vi "WS1050 CAPDAC Setting Updated.vi"(6 "DUT Mask Mode (All)":T1=enum."All", 8 "error in":errorcluster, 9 "C3 Cap DAC":u8=128 caption="B Data In" format="0x%02x", 10 "C2 Cap DAC":u8=128 caption="B Data In" format="0x%02x", 11 "C1 Cap DAC":u8=128 caption="B Data In" format="0x%02x") -> (0 "error out":errorcluster)   [LabVIEW 2012]
uses:
  WS_VCAP Driver 029/Source/WSVCAP Shell/Type Defs/WSVCAP SHL I2C DUT Mask Mode Enum.ctl
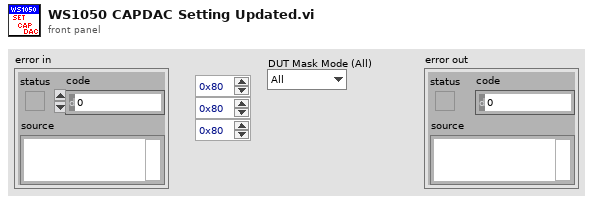
[diagram p1: front panel]
types:
  T1 = typedef "WSVCAP SHL I2C DUT Mask Mode Enum.ctl" = enum16{"Custom", "C1", "C2", "C3", "All"}
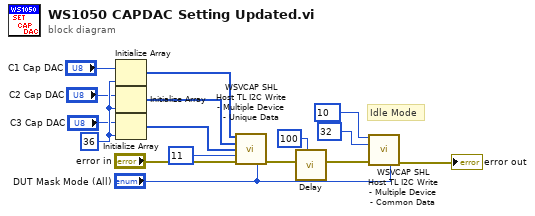
[diagram p0: block diagram]
diagram:
  w16 = 36 ("dimension size")
  # "Idle Mode"
  n1 = Initialize Array("C1 Cap DAC", w16) -> (w2:u8[])
  n2 = Initialize Array("C2 Cap DAC", w16) -> (w3:u8[])
  n3 = Initialize Array("C3 Cap DAC", w16) -> (w1:u8[])
  n4 = call "WSVCAP SHL Host TL I2C Write - Multiple Device - Unique Data.vi"("C1 Data"=w2, "C2 Data"=w3, "C3 Data"=w1, "Sub Address"=u8 11, "error in"="error in", "DUT Mask Mode (All)"="DUT Mask Mode (All)") -> ("error out"=w8:errorcluster)  [unwired: 9 in]
  n5 = call "Delay.vi"("milliseconds to wait"=u32 100, "error in (no error)"=w8) -> ("error out"=w4:errorcluster)  [unwired: 9 in]
  n6 = call "WSVCAP SHL Host TL I2C Write - Multiple Device - Common Data.vi"("Sub Address"=u8 10, "Data Out [U8]"=u8 32 ("Sub Address"), "error in"=w4, "DUT Mask Mode (All)"="DUT Mask Mode (All)") -> ("error out"=→"error out":errorcluster)  [unwired: 11 in]
